vi "CRYPlot Wave Graph.vi"(6 "sOption":string, 7 "pGraph VI In":refnum<vi>, 9 "Flattened Plot Property":string, 10 "Flattened Scale Property":string, 11 "Selected Rows In":i32[](array[numeric])) -> (0 "ItemSyms":i32[](array[numeric]), 1 "Color Info":u32[](array[numeric]), 2 "Curve Name":string[](array[string]), 3 "Selected Rows Out":i32[](array[numeric]))   [LabVIEW 2013]
uses:
  CRYWindow/DataView/Control/CRYGraph Scale.ctl
panel:
  in  "Graph Scale Property":T1={"X Scale.Maximum"=0.0, "X Scale.Minimum"=0.0, "Y0 Scale.Maximum"=0.0, "Y0 Scale.Minimum"=0.0, "Y1 Scale.Maximum"=0.0, "Y1 Scale.Minimum"=0.0, "X Scale.MapMode"=2, "Y1 Scale.MapMode"=2, "Y0 Scale.MapMode"=2, "ScaleFitX"=FALSE, "ScaleFitY"=FALSE, "ScaleFitY 2"=FALSE}
  in  "Plot Settings":T2(array[cluster])
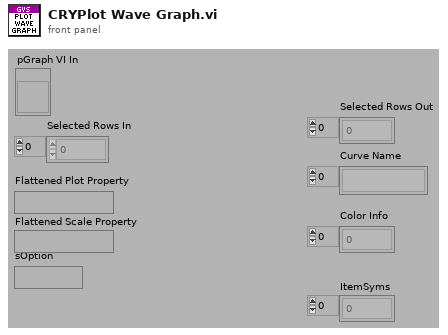
[diagram p1: front panel]
types:
  T1 = typedef "CRYGraph Scale.ctl" = cluster{"X Scale.Maximum":dbl, "X Scale.Minimum":dbl, "Y0 Scale.Maximum":dbl, "Y0 Scale.Minimum":dbl, "Y1 Scale.Maximum":dbl, "Y1 Scale.Minimum":dbl, "X Scale.MapMode":u8, "Y1 Scale.MapMode":u8, "Y0 Scale.MapMode":u8, "ScaleFitX":bool, "ScaleFitY":bool, "ScaleFitY 2":bool}
  T2 = cluster{"Color":u32, "Interpolation":u8, "Point Style":u8, "Line Style":u8, "Point Color":u32, "Line Width":u8, "Bar Plot Style":u8, "Fill To":i16}[]
  T3 = typedef "CRYWaveform Cluster.ctl" = cluster{"Waveform":cluster{"X0":dbl, "dX":dbl, "Y":sgl[]}, "X data":u16, "Y data":u16, "Y axis":u16, "X unit":string, "Y unit":string, "Y dB ref":dbl, "display Y":bool, "display X":bool, "Overload?":bool, "Test Info":string, "Step No.":i32, "Name":string, "protected":bool, "Sqc history":string[], "Signal Channel ID":i32, "Plot Settings":cluster{"Color":u32, "Interpolation":u8, "Point Style":u8, "Line Style":u8, "Point Color":u32, "Line Width":u8, "Bar Plot Style":u8, "Fill To":i16}, "AutoProtect":bool}
  T4 = cluster{"Color":u32, "Interpolation":u8, "Point Style":u8, "Line Style":u8, "Point Color":u32, "Line Width":u8, "Bar Plot Style":u8, "Fill To":i16}
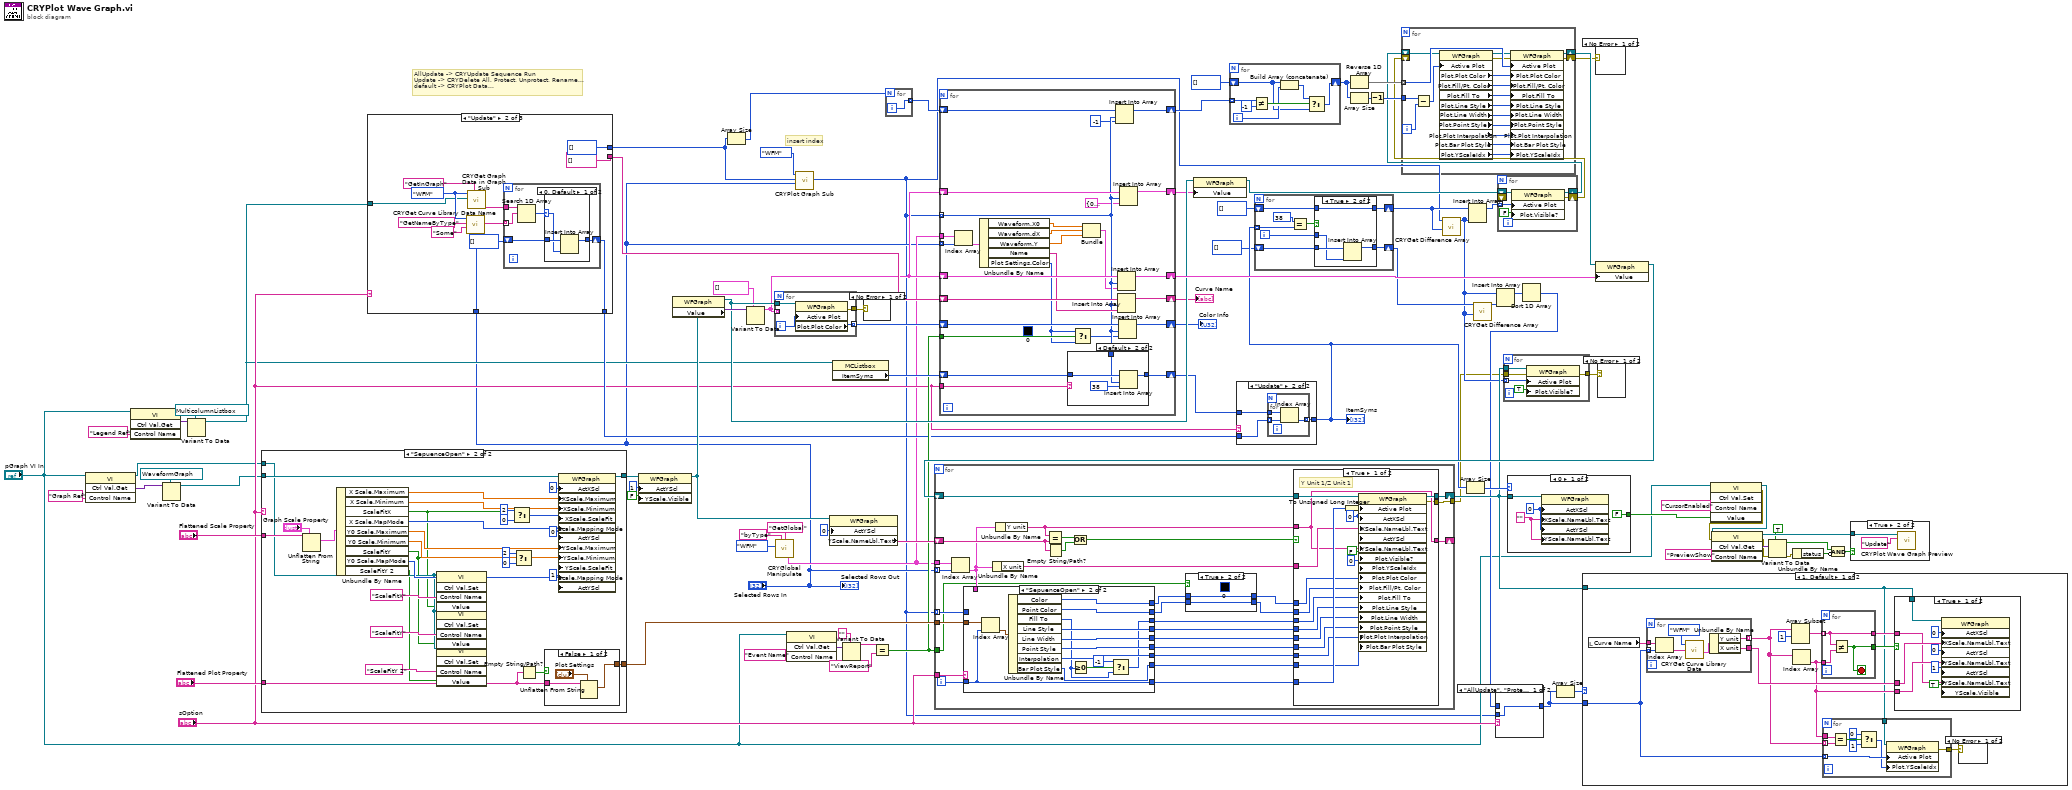
[diagram p0: block diagram]
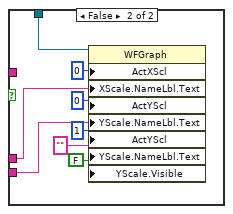
[diagram p5: hidden frame]
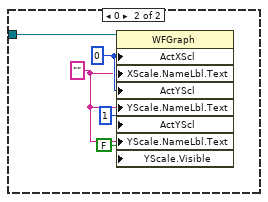
[diagram p6: hidden frame]
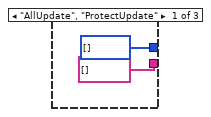
[diagram p9: hidden frame]
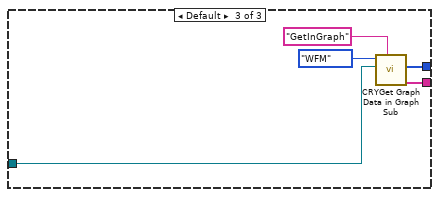
[diagram p11: hidden frame]
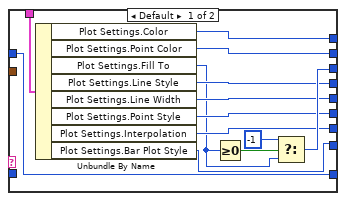
[diagram p15: hidden frame]
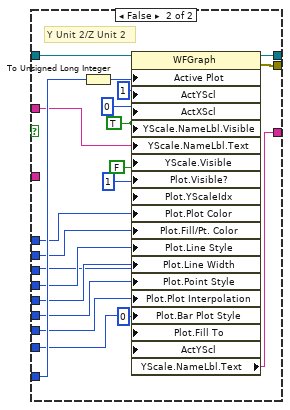
[diagram p16: hidden frame]
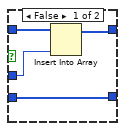
[diagram p17: hidden frame]
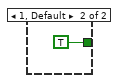
[diagram p19: hidden frame]
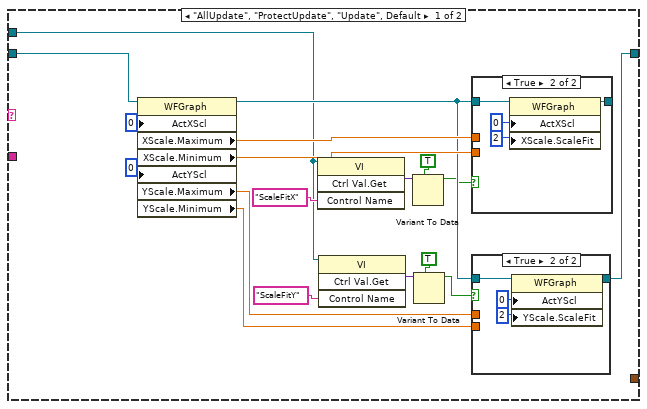
[diagram p20: hidden frame]
diagram:
  # "AllUpdate -> CRYUpdate Sequence Run\nUpdate -> CRYDelete All, Protect, Unprotect, Rename...\ndefault -> CRYPlot Data..."
  # "insert index"
  n1 = invoke class="VI" method="Ctrl Val.Get"(reference="pGraph VI In", "Control Name"="Graph Ref") -> (reference out=w14:refnum<vi>, "Get Control Value Variant"=w16:variant)  [unwired: 2 in, 2 out]
  n2 = invoke class="VI" method="Ctrl Val.Get"(reference="pGraph VI In", "Control Name"="Legend Ref") -> ("Get Control Value Variant"=w12:variant)  [unwired: 2 in, 3 out]
  n3 = Variant To Data(type=refnum<vi> refnum ("WaveGraph Ref"), Variant=w16) -> (data=w15:refnum<vi>)  [unwired: 1 in, 1 out]
  n4 = Variant To Data(type=refnum<vi> refnum ("GMListbox"), Variant=w12) -> (data=w10:refnum<vi>)  [unwired: 1 in, 1 out]
  n5 = case shown="\"SepuenceOpen\"" "sOption" {
    tunnel: w15 -> [w109 w159]
    tunnel: [w105 w158] -> w84
    tunnel: "Flattened Scale Property" -> [_ w148]
    tunnel: "Flattened Plot Property" -> [_ w146]
    tunnel: [_ w145] -> w52
    tunnel: w14 -> [w92 w133]
    frame "AllUpdate", "ProtectUpdate", "Update", Default {
      n6 = property class="WFGraph"(reference=w109, "ActXScl"=0 ("Active X Scale"), "ActYScl"=0 ("Active Y Scale")) -> (reference out=w101:refnum<vi>, "XScale.Maximum"=w103:dbl, "XScale.Minimum"=w108:dbl, "YScale.Maximum"=w107:dbl, "YScale.Minimum"=w106:dbl)  [unwired: 1 in, 1 out]
      n7 = invoke class="VI" method="Ctrl Val.Get"(reference=w92, "Control Name"="ScaleFitX") -> ("Get Control Value Variant"=w96:variant)  [unwired: 2 in, 3 out]
      n8 = invoke class="VI" method="Ctrl Val.Get"(reference=w92, "Control Name"="ScaleFitY") -> ("Get Control Value Variant"=w99:variant)  [unwired: 2 in, 3 out]
      n9 = Variant To Data(type=TRUE, Variant=w96) -> (data=w94:bool)  [unwired: 1 in, 1 out]
      n10 = Variant To Data(type=TRUE, Variant=w99) -> (data=w93:bool)  [unwired: 1 in, 1 out]
      n11 = case shown="True" w94 {
        tunnel: w103 -> [w125 _]
        tunnel: w108 -> [w124 _]
        tunnel: w101 -> [w123 w129]
        tunnel: [w122 w128] -> _
        frame False {
          n12 = property class="WFGraph"(reference=w123, "ActXScl"=0 ("Active X Scale"), "XScale.Maximum"=w125, "XScale.Minimum"=w124, "XScale.ScaleFit"=u8 0 ("X Scale.Scale Fit")) -> (reference out=w122:refnum<vi>)  [unwired: 1 in, 1 out]
        }
        frame True {
          n13 = property class="WFGraph"(reference=w129, "ActXScl"=0 ("Active X Scale"), "XScale.ScaleFit"=u8 2 ("X Scale.Scale Fit")) -> (reference out=w128:refnum<vi>)  [unwired: 1 in, 1 out]
        }
      }
      n14 = case shown="True" w93 {
        tunnel: w101 -> [w115 w119]
        tunnel: [w114 w118] -> w105
        tunnel: w107 -> [w113 _]
        tunnel: w106 -> [w112 _]
        frame False {
          n15 = property class="WFGraph"(reference=w115, "ActYScl"=0 ("Active Y Scale"), "YScale.Maximum"=w113, "YScale.Minimum"=w112, "YScale.ScaleFit"=u8 0 ("Y Scale.Scale Fit")) -> (reference out=w114:refnum<vi>)  [unwired: 1 in, 1 out]
        }
        frame True {
          n16 = property class="WFGraph"(reference=w119, "ActYScl"=0 ("Active Y Scale"), "YScale.ScaleFit"=u8 2 ("Y Scale.Scale Fit")) -> (reference out=w118:refnum<vi>)  [unwired: 1 in, 1 out]
        }
      }
    }
    frame "SepuenceOpen" {
      n17 = Unflatten From String(type="Graph Scale Property", binary string=w148) -> (value=w147:T1)  [unwired: 3 in, 2 out]
      n18 = Unbundle By Name(w147) -> ("X Scale.Maximum"=w144:dbl, "X Scale.Minimum"=w153:dbl, "ScaleFitX"=w132:bool, "X Scale.MapMode"=w156:u8, "Y0 Scale.Maximum"=w154:dbl, "Y0 Scale.Minimum"=w155:dbl, "ScaleFitY"=w131:bool, "Y0 Scale.MapMode"=w157:u8, "ScaleFitY 2"=w130:bool)
      n19 = invoke class="VI" method="Ctrl Val.Set"(reference=w133, "Control Name"="ScaleFitX", "Value"=w132) -> ()  [unwired: 2 in, 5 out]
      n20 = invoke class="VI" method="Ctrl Val.Set"(reference=w133, "Control Name"="ScaleFitY", "Value"=w131) -> ()  [unwired: 2 in, 5 out]
      n21 = invoke class="VI" method="Ctrl Val.Set"(reference=w133, "Control Name"="ScaleFitY 2", "Value"=w130) -> ()  [unwired: 2 in, 5 out]
      n22 = Select(t=u8 2, s=w132, f=u8 0 ("X Scale.Scale Fit")) -> (s? t:f=w138:u8)
      n23 = Select(t=u8 2, s=w131, f=u8 0 ("X Scale.Scale Fit")) -> (s? t:f=w137:u8)
      n24 = Empty String/Path?(string/path=w146) -> (empty?=w150:bool)
      n25 = case shown="False" w150 {
        tunnel: w146 -> [w162 _]
        tunnel: [w160 _] -> w145
        frame False {
          n26 = Unflatten From String(type="Plot Settings", binary string=w162) -> (value=w160:T2)  [unwired: 3 in, 2 out]
        }
        frame True {
        }
      }
      n27 = property class="WFGraph"(reference=w159, "ActXScl"=0 ("Active X Scale"), "XScale.Maximum"=w144, "XScale.Minimum"=w153, "XScale.ScaleFit"=w138, "XScale.Mapping Mode"=w156, "ActYScl"=0 ("Active Y Scale"), "YScale.Maximum"=w154, "YScale.Minimum"=w155, "YScale.ScaleFit"=w137, "YScale.Mapping Mode"=w157, "ActYScl"=1 ("Active Y Scale")) -> (reference out=w158:refnum<vi>)  [unwired: 1 in, 1 out]
    }
  }
  n28 = case shown="\"Update\"" "sOption" {
    tunnel: [i32[] [] ("Rows") i32[] [] ("Rows") w190] -> w3
    tunnel: [string[] [] ("Names Out") string[] [] ("Names Out") w189] -> w80
    tunnel: "Selected Rows In" -> [_ w167 _]
    tunnel: [_ w166 _] -> w40
    tunnel: w10 -> [_ w165 w186]
    frame "AllUpdate", "ProtectUpdate" {
    }
    frame "Update" {
      w169 = enum16{"Curves", "Values", "Results", "WFM"}."WFM" ("Type")
      n29 = call "CRYGet Curve Library Data Name.vi"("nData"=w167, "sOption"="Some", "sAction"="GetNameByType", "Type"=w169) -> ("sNames"=w173:string[])  [unwired: 4 in, 3 out]
      n30 = call "CRYGet Graph Data in Graph Sub.vi"("sOption"="GetInGraph", "Legend Refnum"=w165, "Type In"=w169) -> ("Names Out"=w172:string[])  [unwired: 4 in, 4 out]
      n31 = for {
        tunnel: w172 -> [w178]
        tunnel: w173 -> [w177] mode=indexing
        shift-right: [w179] -> w166
        shift-left: i32[] [] -> [w180]
        n32 = Search 1D Array(1D array=w178, element=w177) -> (index of element=w181:i32)  [unwired: 1 in]
        n33 = case shown="0, Default" w181 {
          selector: w181 -> [w182 _]
          tunnel: w180 -> [w184 w185]
          tunnel: [w183 w185] -> w179
          frame 0, Default {
            n34 = Insert Into Array(array=w184, new element=w182) -> (w183:i32[])  [unwired: 1 in]
          }
          frame -1 {
          }
        }
      }
    }
    frame Default {
      n35 = call "CRYGet Graph Data in Graph Sub.vi"("sOption"="GetInGraph", "Legend Refnum"=w186, "Type In"=enum16{"Curves", "Values", "Results", "WFM"}."WFM" ("Type")) -> ("Names Out"=w189:string[], "Rows"=w190:i32[])  [unwired: 4 in, 3 out]
    }
  }
  n36 = property class="WFGraph"(reference=w84, "ActYScl"=1 ("Active Y Scale"), "YScale.Visible"=FALSE ("Y Scale.Visible")) -> (reference out=w54:refnum<vi>)  [unwired: 1 in, 1 out]
  n37 = property class="WFGraph"(reference=w54) -> (reference out=w79:refnum<vi>, "Value"=w83:variant)  [unwired: 1 in, 1 out]
  n38 = Array Size(array=w3) -> (size(s)=w66:i32)
  n39 = Variant To Data(type=cluster{"xo":dbl, "dx":dbl, dbl[]}[] [] ("appended array"), Variant=w83) -> (data=w74:cluster{"xo":dbl, "dx":dbl, dbl[]}[])  [unwired: 1 in, 1 out]
  n40 = for {
    tunnel: w74 -> [_] mode=indexing
    tunnel: w79 -> [w194]
    tunnel: [w192] -> w81 mode=indexing
    tunnel: [w191] -> w19
    i -> [w193]
    n41 = property class="WFGraph"(reference=w194, "Active Plot"=w193) -> (error out=w191:errorcluster, "Plot.Plot Color"=w192:u32)  [unwired: 1 in, 1 out]
  }
  n42 = call "CRYGlobal Manipulate.vi"("Type"=enum16{"Curves", "Values", "Results", "WFM"}."WFM", "sOption"="byType", "sAction"="GetGlobal") -> ("WFM Out"=w5:T3[])  [unwired: 6 in, 6 out]
  n43 = invoke class="VI" method="Ctrl Val.Get"(reference="pGraph VI In", "Control Name"="Event Name") -> ("Get Control Value Variant"=w48:variant)  [unwired: 2 in, 3 out]
  n44 = call "CRYPlot Graph Sub.vi"("nData2 In"="Selected Rows In", "nData1 In"=w3, "Type"=enum16{"Curves", "Values", "Results", "WFM"}."WFM") -> ("nData Out"=w1:i32[])  [unwired: 8 in]
  n45 = property class="WFGraph"(reference=w54, "ActYScl"=0 ("Active Y Scale")) -> ("YScale.NameLbl.Text"=w53:string)  [unwired: 1 in, 2 out]
  n46 = property class="MCListbox"(reference=w10) -> ("ItemSyms"=w75:i32[])  [unwired: 1 in, 2 out]
  n47 = Variant To Data(type="" ("Control Name"), Variant=w48) -> (data=w46:string)  [unwired: 1 in, 1 out]
  n48 = case shown="No Error" w19 {
    frame No Error {
    }
    frame Error {
    }
  }
  n49 = Equal?(x=w46, y="ViewReport" ("regular expression")) -> (x = y?=w44:bool)
  n50 = for {
    N: w66 -> [_]
    tunnel: [w195] -> w65 mode=indexing
    i -> [w195]
  }
  n51 = for {
    tunnel: w5 -> [w222]
    tunnel: "Selected Rows In" -> [w219] mode=indexing
    shift-right: [w220] -> w82
    shift-left: w74 -> [w221]
    tunnel: w1 -> [w206] mode=indexing
    shift-right: [w213] -> w77
    shift-left: w80 -> [w217]
    shift-right: [w214] -> w39
    shift-left: w81 -> [w215]
    shift-right: [w211] -> w41
    shift-left: w75 -> [w212]
    shift-right: [w209] -> w73
    shift-left: w74 -> [w210]
    shift-right: [w207] -> w57
    shift-left: w65 -> [w208]
    tunnel: w44 -> [w199]
    tunnel: "sOption" -> [w197]
    (unwired) u32 0
    n52 = Index Array(array=w222, index=w219) -> (element=w218:T3)
    n53 = Unbundle By Name(w218) -> ("Waveform.X0"=w204:dbl, "Waveform.dX"=w203:dbl, "Waveform.Y"=w202:sgl[], "Name"=w216:string, "Plot Settings.Color"=w196:u32)
    n54 = case shown="Default" w197 {
      tunnel: w212 -> [w223 w226]
      tunnel: [w223 w225] -> w211
      tunnel: w206 -> [_ w224]
      frame "AllUpdate", "ProtectUpdate", "Update" {
      }
      frame Default {
        n55 = Insert Into Array(array=w226, index=w224, new element=38) -> (w225:i32[])
      }
    }
    n56 = Select(t=w196, s=w199, f=w196) -> (s? t:f=w198:u32)
    n57 = Bundle("X0"=w204, "dX"=w203, "Y"=w202) -> (w201:cluster{"X0":dbl, "dX":dbl, "Y":sgl[]})  [unwired: 1 in]
    n58 = Insert Into Array(array=w208, index=w206, new element=-1 ("new element/subarray")) -> (w207:i32[])
    n59 = Insert Into Array(array=w221, index=w206, new element=w201) -> (w220:cluster{"xo":dbl, "dx":dbl, dbl[]}[])
    n60 = Insert Into Array(array=w217, index=w206, new element=w216) -> (w213:string[])
    n61 = Insert Into Array(array=w215, index=w206, new element=w198) -> (w214:u32[])
    n62 = Insert Into Array(array=w210, index=w206, new element=cluster{"xo":dbl, "dx":dbl, dbl[]} {"xo"=0.0, "dx"=0.0, []}) -> (w209:cluster{"xo":dbl, "dx":dbl, dbl[]}[])
  }
  "Curve Name" <- w77
  "Color Info" <- w39
  n63 = property class="WFGraph"(reference=w79, "Value"=w73) -> (reference out=w78:refnum<vi>)  [unwired: 1 in, 1 out]
  n64 = for {
    tunnel: w57 -> [w234] mode=indexing
    shift-right: [w230] -> w62
    shift-left: i32[] [] ("Selected Rows In") -> [w228]
    i -> [w229]
    n65 = Not Equal?(x=w234, y=-1) -> (x != y?=w232:bool)
    n66 = Build Array (concatenate)(w228, w229) -> (w231:i32[])
    n67 = Select(t=w231, s=w232, f=w228) -> (s? t:f=w230:i32[])
  }
  n68 = case shown="\"Update\"" "sOption" {
    tunnel: w40 -> [_ w237]
    tunnel: w41 -> [w235 w238]
    tunnel: [w235 w236] -> w37
    frame Default {
    }
    frame "Update" {
      n69 = for {
        tunnel: w238 -> [w241]
        tunnel: w237 -> [w240] mode=indexing
        tunnel: [w239] -> w236 mode=indexing
        n70 = Index Array(array=w241, index=w240) -> (element=w239:i32)
      }
    }
  }
  "ItemSyms" <- w37
  n71 = for {
    tunnel: w37 -> [w248] mode=indexing
    shift-right: [w247] -> w43
    shift-left: i32[] [] ("Selected Rows In") -> [w246]
    shift-right: [w242] -> w32
    shift-left: i32[] [] ("Selected Rows In") -> [w243]
    i -> [w245]
    n72 = Equal?(x=38, y=w248) -> (x = y?=w244:bool)
    n73 = case shown="True" w244 {
      tunnel: [w252 w254] -> w247
      tunnel: w246 -> [w253 w254]
      tunnel: w245 -> [w251 w256]
      tunnel: w243 -> [w250 w257]
      tunnel: [w250 w255] -> w242
      frame False {
        n74 = Insert Into Array(array=w253, new element=w251) -> (w252:i32[])  [unwired: 1 in]
      }
      frame True {
        n75 = Insert Into Array(array=w257, new element=w256) -> (w255:i32[])  [unwired: 1 in]
      }
    }
  }
  n76 = Reverse 1D Array(array=w62) -> (reversed array=w61:i32[])
  n77 = Array Size(array=w62) -> (size(s)=w63:i32)
  n78 = Decrement(x=w63) -> (x-1=w64:i32)
  n79 = call "CRYGet Difference Array.vi"("Array 2"=w43, "Array 1"=w1) -> ("Diff Out"=w31:i32[])  [unwired: 8 in, 1 out]
  n80 = Array Size(array=w37) -> (size(s)=w91:i32)
  n81 = Insert Into Array(array=w43, new element=w31) -> (w67:i32[])  [unwired: 1 in]
  n82 = call "CRYGet Difference Array.vi"("Array 2"=w31, "Array 1"=w32) -> ("Diff Out"=w35:i32[])  [unwired: 8 in, 1 out]
  n83 = Insert Into Array(array=w31, new element=w35) -> (w34:i32[])  [unwired: 1 in]
  n84 = for {
    tunnel: w67 -> [w260] mode=indexing
    shift-right: [w259] -> w59
    shift-left: w78 -> [w262]
    shift-right: [w258] -> w42
    shift-left: _ -> [_]
    n85 = property class="WFGraph"(reference=w262, "Active Plot"=w260, "Plot.Visible?"=FALSE ("Plot.Visible")) -> (reference out=w259:refnum<vi>, error out=w258:errorcluster)  [unwired: 1 in]
  }
  n86 = for {
    tunnel: w61 -> [w274] mode=indexing
    shift-right: [w272] -> w58
    shift-left: w59 -> [w273]
    tunnel: w64 -> [w269]
    shift-right: [w265] -> w51
    shift-left: w42 -> [_]
    i -> [w268]
    n87 = Subtract(x=w269, y=w268) -> (x-y=w267:i32)
    n88 = property class="WFGraph"(reference=w273, "Active Plot"=w267) -> (reference out=w271:refnum<vi>, error out=w266:errorcluster, "Plot.Plot Color"=w280:u32, "Plot.Fill/Pt. Color"=w279:u32, "Plot.Fill To"=w278:i16, "Plot.Line Style"=w277:u8, "Plot.Line Width"=w276:u8, "Plot.Point Style"=w275:u8, "Plot.Plot Interpolation"=w270:u8, "Plot.Bar Plot Style"=w264:u8, "Plot.YScaleIdx"=w263:u32)  [unwired: 1 in]
    n89 = property class="WFGraph"(reference=w271, error in=w266, "Active Plot"=w274, "Plot.Plot Color"=w280, "Plot.Fill/Pt. Color"=w279, "Plot.Fill To"=w278, "Plot.Line Style"=w277, "Plot.Line Width"=w276, "Plot.Point Style"=w275, "Plot.Plot Interpolation"=w270, "Plot.Bar Plot Style"=w264, "Plot.YScaleIdx"=w263) -> (reference out=w272:refnum<vi>, error out=w265:errorcluster)
  }
  n90 = Sort 1D Array(array=w34) -> (sorted array=w28:i32[])
  n91 = case shown="\"AllUpdate\", \"ProtectUpdate\", \"SepuenceOpen\"" "sOption" {
    tunnel: [w281 w282] -> w27
    tunnel: w1 -> [w281 _]
    tunnel: w28 -> [_ w282]
    frame "AllUpdate", "ProtectUpdate", "SepuenceOpen" {
    }
    frame Default {
    }
  }
  n92 = Array Size(array=w27) -> (size(s)=w30:i32)
  n93 = case shown="No Error" w51 {
    frame No Error {
    }
    frame Error {
    }
  }
  n94 = property class="WFGraph"(reference=w58, "Value"=w82) -> (reference out=w56:refnum<vi>)  [unwired: 1 in, 1 out]
  n95 = for {
    tunnel: "Selected Rows In" -> [w311] mode=indexing
    tunnel: w5 -> [w310]
    tunnel: w52 -> [w305]
    tunnel: "sOption" -> [w306]
    shift-right: [w307] -> w36
    shift-left: w56 -> [w296]
    tunnel: w1 -> [w295] mode=indexing
    shift-right: [w293] -> _
    shift-left: w53 -> [w299]
    tunnel: w44 -> [w285]
    tunnel: [w283] -> w20
    i -> [w300]
    n96 = Index Array(array=w310, index=w311) -> (element=w298:T3)
    n97 = case shown="\"SepuenceOpen\"" w306 {
      tunnel: w305 -> [_ w338]
      tunnel: [w328 w332] -> w289
      tunnel: [w317 w331] -> w288
      tunnel: [w327 w333] -> w284
      tunnel: [w326 w342] -> w304
      tunnel: [w325 w341] -> w303
      tunnel: [w324 w340] -> w302
      tunnel: [w323 w339] -> w301
      tunnel: w298 -> [w322 _]
      tunnel: w300 -> [_ w330]
      tunnel: [w318 w330] -> w294
      tunnel: w295 -> [w318 _]
      tunnel: [w316 w329] -> w290
      frame Default {
        n98 = Unbundle By Name(w322) -> ("Plot Settings.Color"=w328:u32, "Plot Settings.Point Color"=w317:u32, "Plot Settings.Fill To"=w319:i16, "Plot Settings.Line Style"=w326:u8, "Plot Settings.Line Width"=w325:u8, "Plot Settings.Point Style"=w324:u8, "Plot Settings.Interpolation"=w323:u8, "Plot Settings.Bar Plot Style"=w316:u8)
        n99 = Greater Or Equal To 0?(x=w319) -> (x >= 0?=w321:bool)
        n100 = Select(t=i16 -1 ("Fill To"), s=w321, f=w319) -> (s? t:f=w327:i16)
      }
      frame "SepuenceOpen" {
        n101 = Index Array(array=w338, index=w330) -> (element=w337:T4)
        n102 = Unbundle By Name(w337) -> ("Color"=w332:u32, "Point Color"=w331:u32, "Fill To"=w334:i16, "Line Style"=w342:u8, "Line Width"=w341:u8, "Point Style"=w340:u8, "Interpolation"=w339:u8, "Bar Plot Style"=w329:u8)
        n103 = Greater Or Equal To 0?(x=w334) -> (x >= 0?=w336:bool)
        n104 = Select(t=i16 -1 ("Fill To"), s=w336, f=w334) -> (s? t:f=w333:i16)
      }
    }
    n105 = Unbundle By Name(w298) -> ("X unit"=w297:string)
    n106 = Unbundle By Name(w298) -> ("Y unit"=w308:string)
    n107 = Equal?(x=w308, y=w299) -> (x = y?=w291:bool)
    n108 = Empty String/Path?(string/path=w299) -> (empty?=w292:bool)
    n109 = Or(x=w291, y=w292) -> (x .or. y?=w309:bool)
    n110 = case shown="True" w285 {
      tunnel: [w313 w315] -> w287
      tunnel: w289 -> [w313 w315]
      tunnel: w288 -> [w312 w314]
      tunnel: [w312 w314] -> w286
      frame False {
      }
      frame True {
        (unwired) u32 0
      }
    }
    n111 = case shown="True" w309 {
      tunnel: w297 -> [w350 _]
      tunnel: w296 -> [w360 w380]
      tunnel: w294 -> [w359 w381]
      tunnel: w308 -> [w345 w366]
      tunnel: [w358 w379] -> w307
      tunnel: w287 -> [w357 w378]
      tunnel: w286 -> [w356 w377]
      tunnel: w284 -> [w355 w362]
      tunnel: w304 -> [w354 w376]
      tunnel: w303 -> [w353 w375]
      tunnel: w302 -> [w352 w374]
      tunnel: w301 -> [w351 w373]
      tunnel: [w345 w364] -> w293
      tunnel: w290 -> [w344 w363]
      tunnel: [w343 w361] -> w283
      frame True {
        w347 = 0 ("Active X Scale")
        # "Y Unit 1/Z Unit 1"
        n112 = To Unsigned Long Integer(number=w359) -> (unsigned 32bit integer=w346:u32)
        n113 = property class="WFGraph"(reference=w360, "Active Plot"=w346, "ActXScl"=w347, "XScale.NameLbl.Text"=w350, "ActYScl"=w347, "YScale.NameLbl.Text"=w345, "Plot.Visible?"=FALSE ("Plot.Visible"), "Plot.YScaleIdx"=u32 0 ("Plot.Y Scale Index"), "Plot.Plot Color"=w357, "Plot.Fill/Pt. Color"=w356, "Plot.Fill To"=w355, "Plot.Line Style"=w354, "Plot.Line Width"=w353, "Plot.Point Style"=w352, "Plot.Plot Interpolation"=w351, "Plot.Bar Plot Style"=w344) -> (reference out=w358:refnum<vi>, error out=w343:errorcluster)  [unwired: 1 in]
      }
      frame False {
        w369 = TRUE ("Y Scale.Name Label.Visible")
        # "Y Unit 2/Z Unit 2"
        n114 = To Unsigned Long Integer(number=w381) -> (unsigned 32bit integer=w368:u32)
        n115 = property class="WFGraph"(reference=w380, "Active Plot"=w368, "ActYScl"=1 ("Active Y Scale"), "ActXScl"=0 ("Active X Scale"), "YScale.NameLbl.Visible"=w369, "YScale.NameLbl.Text"=w366, "YScale.Visible"=w369, "Plot.Visible?"=FALSE ("Plot.Visible"), "Plot.YScaleIdx"=u32 1 ("Plot.Y Scale Index"), "Plot.Plot Color"=w378, "Plot.Fill/Pt. Color"=w377, "Plot.Line Style"=w376, "Plot.Line Width"=w375, "Plot.Point Style"=w374, "Plot.Plot Interpolation"=w373, "Plot.Bar Plot Style"=w363, "Plot.Fill To"=w362, "ActYScl"=0 ("Active Y Scale")) -> (reference out=w379:refnum<vi>, error out=w361:errorcluster, "YScale.NameLbl.Text"=w364:string)  [unwired: 1 in]
      }
    }
  }
  n116 = for {
    tunnel: w36 -> [w386]
    tunnel: w31 -> [w384] mode=indexing
    tunnel: [w383] -> w38
    tunnel: w20 -> [w382]
    n117 = property class="WFGraph"(reference=w386, error in=w382, "Active Plot"=w384, "Plot.Visible?"=TRUE ("Plot.Visible")) -> (error out=w383:errorcluster)  [unwired: 1 out]
  }
  n118 = case shown="0" w91 {
    tunnel: w36 -> [w388 _]
    tunnel: [FALSE TRUE] -> w89
    frame 0 {
      w390 = 0 ("Active X Scale")
      w389 = "" ("X Scale.Name Label.Text")
      n119 = property class="WFGraph"(reference=w388, "ActXScl"=w390, "XScale.NameLbl.Text"=w389, "ActYScl"=w390, "YScale.NameLbl.Text"=w389) -> ()  [unwired: 1 in, 2 out]
    }
    frame 1, Default {
    }
  }
  n120 = case shown="1, Default" w30 {
    tunnel: w27 -> [w394 _]
    tunnel: w36 -> [w392 w441]
    frame 1, Default {
      n121 = local read "Curve Name"() -> (w402:string[])
      n122 = for {
        tunnel: w402 -> [w436]
        tunnel: w394 -> [w437] mode=indexing
        tunnel: [w433] -> w396 mode=indexing
        tunnel: [w432] -> w398
        n123 = Index Array(array=w436, index=w437) -> (element=w435:string)
        n124 = call "CRYGet Curve Library Data.vi"("Type"=enum16{"Curves", "Values", "Results", "WFM"}."WFM", "Data Name"=w435) -> ("Wave"=w431:T3)  [unwired: 4 out]
        n125 = Unbundle By Name(w431) -> ("Y unit"=w433:string, "X unit"=w432:string)
      }
      n126 = Array Subset(array=w396, index=1) -> (w400:string[])  [unwired: 1 in]
      n127 = Index Array(array=w396) -> (element=w395:string)  [unwired: 1 in]
      n128 = for {
        tunnel: w400 -> [w428] mode=indexing
        tunnel: w395 -> [w430]
        tunnel: [w429] -> w399
        tunnel: [w428] -> w397
        stop <- w429 stop-if-true
        n129 = Not Equal?(x=w428, y=w430) -> (x != y?=w429:bool)
      }
      n130 = for {
        tunnel: w394 -> [w411] mode=indexing
        tunnel: w396 -> [w409] mode=indexing
        tunnel: w395 -> [w410]
        tunnel: w392 -> [w404]
        tunnel: [w403] -> w393
        n131 = Equal?(x=w410, y=w409) -> (x = y?=w408:bool)
        n132 = Select(t=u32 0 ("Plot.Y Scale Index"), s=w408, f=u32 1 ("Plot.Y Scale Index")) -> (s? t:f=w405:u32)
        n133 = property class="WFGraph"(reference=w404, "Active Plot"=w411, "Plot.YScaleIdx"=w405) -> (error out=w403:errorcluster)  [unwired: 1 in, 1 out]
      }
      n134 = case shown="True" w399 {
        tunnel: w392 -> [w417 w425]
        tunnel: w395 -> [w415 w423]
        tunnel: w398 -> [w414 w421]
        tunnel: w397 -> [w412 _]
        frame True {
          n135 = property class="WFGraph"(reference=w417, "ActXScl"=0 ("Active X Scale"), "XScale.NameLbl.Text"=w414, "ActYScl"=0 ("Active X Scale"), "YScale.NameLbl.Text"=w415, "ActYScl"=1 ("Active Y Scale"), "YScale.NameLbl.Text"=w412, "YScale.Visible"=TRUE ("Y Scale.Visible")) -> ()  [unwired: 1 in, 2 out]
        }
        frame False {
          n136 = property class="WFGraph"(reference=w425, "ActXScl"=0 ("Active X Scale"), "XScale.NameLbl.Text"=w421, "ActYScl"=0 ("Active X Scale"), "YScale.NameLbl.Text"=w423, "ActYScl"=1 ("Active Y Scale"), "YScale.NameLbl.Text"="" ("Y Scale.Name Label.Text"), "YScale.Visible"=FALSE ("Y Scale.Visible")) -> ()  [unwired: 1 in, 2 out]
        }
      }
      n137 = case shown="No Error" w393 {
        frame No Error {
        }
        frame Error {
        }
      }
    }
    frame 0 {
      w442 = 0 ("Active X Scale")
      w439 = "" ("X Scale.Name Label.Text")
      n138 = property class="WFGraph"(reference=w441, "ActXScl"=w442, "XScale.NameLbl.Text"=w439, "ActYScl"=w442, "YScale.NameLbl.Text"=w439, "ActYScl"=1 ("Active Y Scale"), "YScale.NameLbl.Text"=w439, "YScale.Visible"=FALSE ("Y Scale.Visible")) -> ()  [unwired: 1 in, 2 out]
    }
  }
  n139 = case shown="No Error" w38 {
    frame No Error {
    }
    frame Error {
    }
  }
  n140 = invoke class="VI" method="Ctrl Val.Set"(reference="pGraph VI In", "Control Name"="CursorEnabled", "Value"=w89) -> (reference out=w71:refnum<vi>, error out=w26:errorcluster)  [unwired: 2 in, 3 out]
  n141 = invoke class="VI" method="Ctrl Val.Get"(reference=w71, error in=w26, "Control Name"="PreviewShow") -> (reference out=w70:refnum<vi>, error out=w25:errorcluster, "Get Control Value Variant"=w69:variant)  [unwired: 1 in, 1 out]
  n142 = Variant To Data(error in=w25, type=TRUE, Variant=w69) -> (data=w23:bool, error out=w24:errorcluster)
  n143 = Unbundle By Name(w24) -> ("status"=w22:bool)
  n144 = Compound Arithmetic op=AND(w23, invert w22) -> (w21:bool)
  n145 = case shown="True" w21 {
    tunnel: w70 -> [_ w444]
    frame False {
    }
    frame True {
      n146 = call "CRYPlot Wave Graph Preview.vi"("sOption"="Update", "Graph VI Ref"=w444) -> ()  [unwired: 10 in]
    }
  }
  "Selected Rows Out" <- "Selected Rows In"
